vi "Experiment and Experimenter.vi"() -> ()   [LabVIEW 2012]
doc: "SciScan 1.2 160622"
panel:
  in  "Experiment and Experimenter Details":T1
  # "Experiment"
  # "Experimenter"
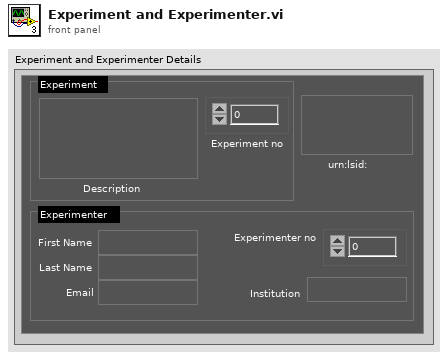
[diagram p1: front panel]
types:
  T1 = cluster{"Experimenter no":u32, "First Name":string, "Experiment no":u32, "urn:lsid: ":string, "Description":string, "Last Name":string, "Email":string, "Institution":string}
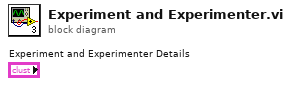
[diagram p0: block diagram]
diagram:
